vi "SetTagsUnits.vi"(8 "error in (no error)":errorcluster, 10 "Tags_Units":T1 {"EAQtagProps"."TagFunc" format="%08x"; "EAQtagProps"."RangeL" format="%.2f"; "EAQtagProps"."RangeH" format="%.2f"; "WAQtagProps"."TagFunc" format="%08x"; "WAQtagProps"."RangeL" format="%.2f"; "WAQtagProps"."RangeH" format="%.2f"; "PAQtagProps"."TagFunc" format="%08x"; "PAQtagProps"."RangeL" format="%.2f"; "PAQtagProps"."RangeH" format="%.2f"}, 11 "Gviewer in":refnum<class "Gviewer.lvclass">) -> (0 "error out":errorcluster, 3 "Gviewer out":refnum<class "Gviewer.lvclass">)   [LabVIEW 2020, in "Sgraph_lib_V1.lvlib" / "Gviewer.lvclass"]
doc: "Write all TAGs and Tag attributes to Gviewer"
uses:
  Gviewer.lvclass
  FAMM/controls/Typedef_Gviewer_TagsUnits.ctl
  Common/controls/typedef_com_TagProp.ctl
  DBAL/controls/DBAL_TAGpropEdit.ctl
  Gviewer.lvclass/Gviewer.ctl
  Builds/Sgraph_lib_V1.lvlib
  FAMM/FAMM.lvclass
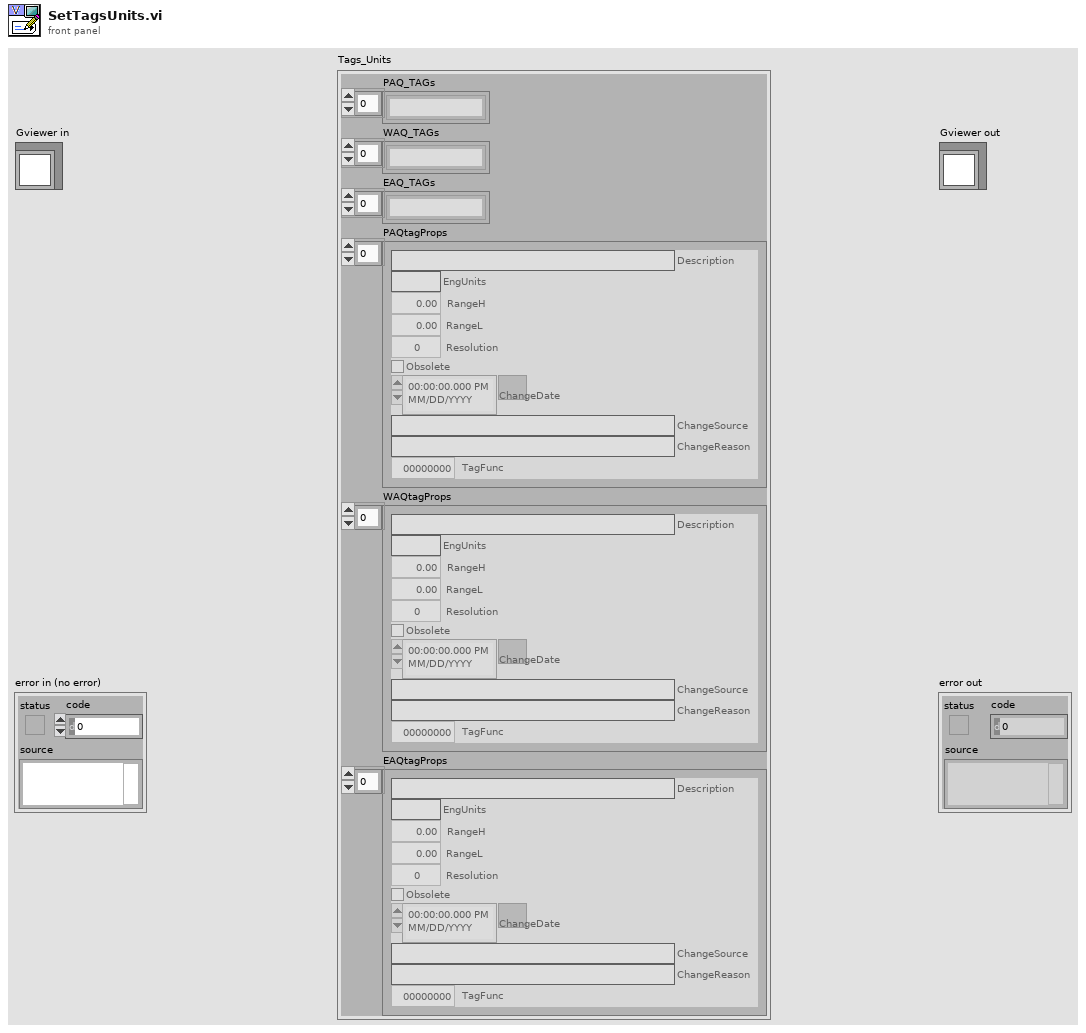
[diagram p1: front panel]
types:
  T1 = typedef "Sgraph_lib_V1.lvlib/FAMM.lvclass/Typedef_Gviewer_TagsUnits.ctl" = cluster{"PAQ_TAGs":string[], "WAQ_TAGs":string[], "EAQ_TAGs":string[], "PAQtagProps":T2[], "WAQtagProps":T2[], "EAQtagProps":T2[]}
  T2 = typedef "Sgraph_lib_V1.lvlib/typedef_com_TagProp.ctl" = cluster{"Description":string, "EngUnits":string, "RangeH":dbl, "RangeL":dbl, "Resolution":i32, "Obsolete":bool, "ChangeDate":timestamp, "ChangeSource":string, "ChangeReason":string, "TagFunc":u32}
  T3 = typedef "Sgraph_lib_V1.lvlib/DBAL_TAGpropEdit.ctl" = cluster{"TAG":string, "Qtype":string, "TAGprop":T2}
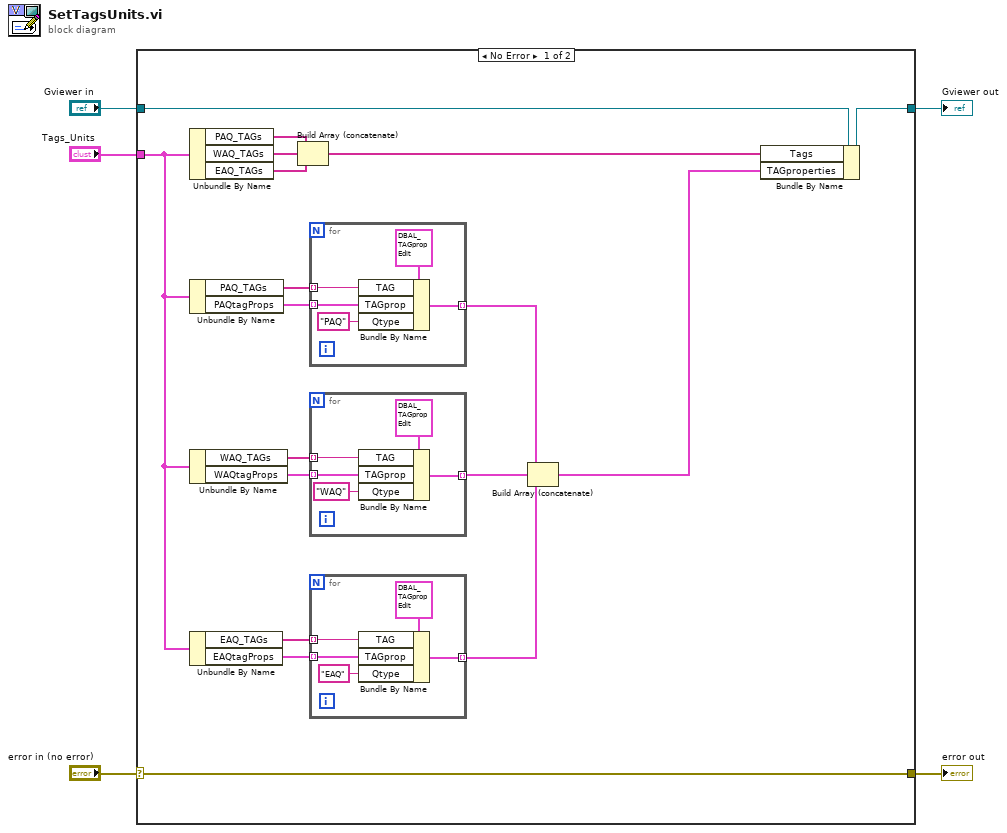
[diagram p0: block diagram]
diagram:
  n1 = case shown="No Error" "error in (no error)" {
    selector: "error in (no error)" -> [w23 w40]
    tunnel: [w23 w40] -> w4
    tunnel: [w7 w39] -> w2
    tunnel: "Gviewer in" -> [w6 w39]
    tunnel: "Tags_Units" -> [w12 _]
    frame No Error {
      n2 = Unbundle By Name(w12) -> ("PAQ_TAGs"=w21:string[], "WAQ_TAGs"=w22:string[], "EAQ_TAGs"=w20:string[])
      n3 = Unbundle By Name(w12) -> ("PAQ_TAGs"=w18:string[], "PAQtagProps"=w17:T2[])
      n4 = Unbundle By Name(w12) -> ("WAQ_TAGs"=w15:string[], "WAQtagProps"=w16:T2[])
      n5 = Unbundle By Name(w12) -> ("EAQ_TAGs"=w14:string[], "EAQtagProps"=w13:T2[])
      n6 = Build Array (concatenate)(w21, w22, w20) -> (w19:string[])
      n7 = for {
        tunnel: w18 -> [w37] mode=indexing
        tunnel: w17 -> [w36] mode=indexing
        tunnel: [w34] -> w11 mode=indexing
        n8 = Bundle By Name(cluster=T3 {"TAG"="", "Qtype"="", "TAGprop"={"Description"="", "EngUnits"="", "RangeH"=0.0, "RangeL"=0.0, "Resolution"=0, "Obsolete"=FALSE, "ChangeDate"=timestamp(0 s since 1904-01-01), "ChangeSource"="", "ChangeReason"="", "TagFunc"=0}} ("TAGpropertyEdit"), "TAG"=w37, "TAGprop"=w36, "Qtype"="PAQ") -> (w34:T3)
      }
      n9 = for {
        tunnel: w15 -> [w32] mode=indexing
        tunnel: w16 -> [w31] mode=indexing
        tunnel: [w29] -> w10 mode=indexing
        n10 = Bundle By Name(cluster=T3 {"TAG"="", "Qtype"="", "TAGprop"={"Description"="", "EngUnits"="", "RangeH"=0.0, "RangeL"=0.0, "Resolution"=0, "Obsolete"=FALSE, "ChangeDate"=timestamp(0 s since 1904-01-01), "ChangeSource"="", "ChangeReason"="", "TagFunc"=0}} ("TAGpropertyEdit"), "TAG"=w32, "TAGprop"=w31, "Qtype"="WAQ") -> (w29:T3)
      }
      n11 = for {
        tunnel: w14 -> [w27] mode=indexing
        tunnel: w13 -> [w26] mode=indexing
        tunnel: [w24] -> w9 mode=indexing
        n12 = Bundle By Name(cluster=T3 {"TAG"="", "Qtype"="", "TAGprop"={"Description"="", "EngUnits"="", "RangeH"=0.0, "RangeL"=0.0, "Resolution"=0, "Obsolete"=FALSE, "ChangeDate"=timestamp(0 s since 1904-01-01), "ChangeSource"="", "ChangeReason"="", "TagFunc"=0}} ("TAGpropertyEdit"), "TAG"=w27, "TAGprop"=w26, "Qtype"="EAQ") -> (w24:T3)
      }
      n13 = Build Array (concatenate)(w11, w10, w9) -> (w8:T3[])
      n14 = Bundle By Name(cluster=w6, "Tags"=w19, "TAGproperties"=w8) -> (w7:refnum<class "Gviewer.lvclass">)
    }
    frame Error {
    }
  }
  "error out" <- w4
  "Gviewer out" <- w2
